vi "Reset Image Array Position.vi"(8 "error in (no error)":errorcluster, 10 "Label array":refnum<vi>[](array[refnum]), 11 "Image ref array":refnum<vi>[](array[refnum])) -> (0 "error in (no error)":errorcluster)   [LabVIEW 2019, in "ZenGage v3.0 UI.lvclass"]
uses:
  ZenGage v3.0 UI.lvclass
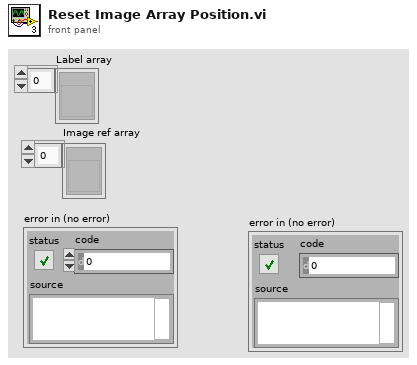
[diagram p1: front panel]
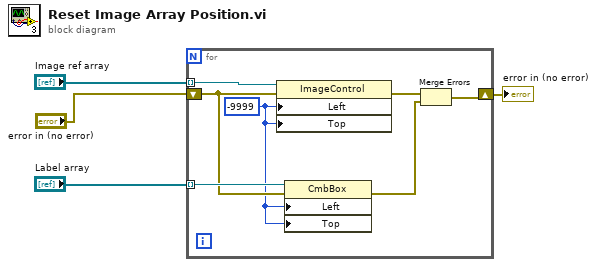
[diagram p0: block diagram]
diagram:
  n1 = for {
    tunnel: "Image ref array" -> [w11] mode=indexing
    shift-right: [w5] -> w2
    shift-left: "error in (no error)" -> [w9]
    tunnel: "Label array" -> [w10] mode=indexing
    w8 = -9999 ("Position:Left")
    n2 = property class="ImageControl"(reference=w11, error in=w9, "Left"=w8, "Top"=w8) -> (error out=w7:errorcluster)  [unwired: 1 out]
    n3 = property class="CmbBox"(reference=w10, error in=w9, "Left"=w8, "Top"=w8) -> (error out=w6:errorcluster)  [unwired: 1 out]
    n4 = Merge Errors(w7, w6) -> (w5:errorcluster)
  }
  "error in (no error)" <- w2
